vi "IsAnyOfType.vi"(8 "error in":errorcluster, 9 "Message Type":string, 10 "Any":T1, 11 "gRPCid in":T2) -> (0 "error out":errorcluster, 1 "Is Type":bool, 3 "gRPCid":T2)   [LabVIEW 2019, in "gprc-lvsupport.lvlib"]
uses:
  gprc-lvsupport.lvlib
  Shared/grpcId.ctl
  Shared/Any.ctl
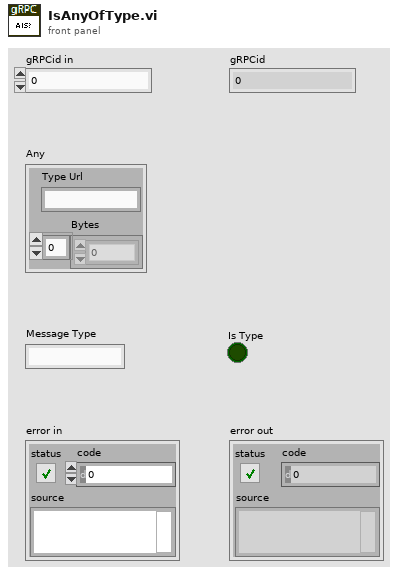
[diagram p1: front panel]
types:
  T1 = typedef "gprc-lvsupport.lvlib/Any.ctl" = cluster{"Type Url":string, "Bytes":u8[]}
  T2 = typedef "gprc-lvsupport.lvlib/grpcId.ctl" = u64
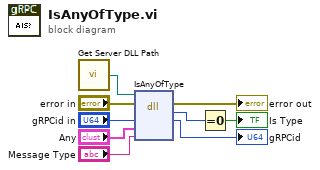
[diagram p0: block diagram]
diagram:
  n1 = call "Get Server DLL Path.vi"() -> ("Server dll path"=w7:path)
  n2 = dll-call lib="?" fn="IsAnyOfType"(path in=w7, error in="error in", "gRPCId"="gRPCid in", "any"="Any", "messageType"="Message Type") -> (error out=→"error out":errorcluster, "return type"=w3:i32, "gRPCId"=→"gRPCid":u64)  [unwired: 3 in, 1 out]
  n3 = Equal To 0?(x=w3) -> (x = 0?=→"Is Type":bool)
